vi "Set Read Position.vi"(8 "error in (no error)":errorcluster, 9 "Relative? (F)":bool, 10 "Offset":i64, 11 "FileStream in":refnum<class "FileStream.lvclass">) -> (0 "error out":errorcluster, 3 "FileStream out":refnum<class "FileStream.lvclass">)   [LabVIEW 2020, in "IO.lvlib" / "FileStream.lvclass"]
uses:
  FileStream.lvclass
  FileStream.lvclass/FileStream.ctl
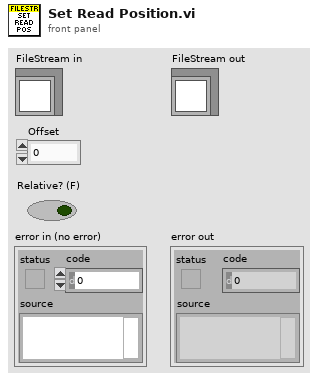
[diagram p1: front panel]
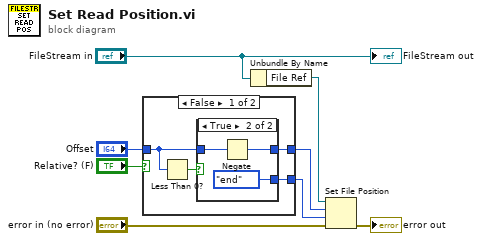
[diagram p0: block diagram]
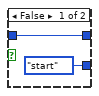
[diagram p2: hidden frame]
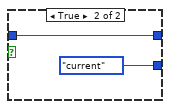
[diagram p3: hidden frame]
diagram:
  n1 = case shown="False" "Relative? (F)" {
    tunnel: "Offset" -> [w11 w19]
    tunnel: [w10 enum16{"start", "end", "current"}."current" ("from (0:start)")] -> w3
    tunnel: [w9 w19] -> w2
    frame False {
      n2 = Less Than 0?(x=w11) -> (x < 0?=w12:bool)
      n3 = case shown="True" w12 {
        tunnel: w11 -> [w14 w17]
        tunnel: [enum16{"start", "end", "current"}."start" ("from (0:start)") enum16{"start", "end", "current"}."end" ("from (0:start)")] -> w10
        tunnel: [w14 w15] -> w9
        frame False {
        }
        frame True {
          n4 = Negate(x=w17) -> (-x=w15:i64)
        }
      }
    }
    frame True {
    }
  }
  n5 = Unbundle By Name("FileStream in") -> ("File Ref"=w5:refnum<file>)
  n6 = Set File Position(offset (in bytes) (0)=w2, refnum=w5, from (0:start)=w3, error in="error in (no error)") -> (error out=→"error out":errorcluster)  [unwired: 1 out]
  "FileStream out" <- "FileStream in"
